vi "通信并与其他模块交互 (子VI).vi"() -> ()   [LabVIEW 2016, in "质控单元.lvlib"]
uses:
  <vilib>/Plasmionique/MB Master/MB_Master_TCP/MB_Master_TCP.lvclass
  C:/Program Files (x86)/National Instruments/LabVIEW 2016/vi.lib/Plasmionique/MB Master/MB_Master/MB_Master.lvclass
  <vilib>/Plasmionique/MB Master/MB_Master/MB_Master.lvclass
  <vilib>/Plasmionique/MB Master/MB Master.lvlib
  <vilib>/Utility/config.llb/NI_LVConfig.lvlib
panel:
  out "CODCr测量状态":u16[](array[numeric])
  out "CODMn测量状态":u16[](array[numeric])
  out "总氮测量状态":u16[](array[numeric])
  out "总磷测量状态":u16[](array[numeric])
  out "氨氮测量状态":u16[](array[numeric])
  out "通讯状态":bool
  out "待处理插入数量":i32
  out "元素":cluster{"命令":string}[](array[cluster])
  out "队列中元素数量":i32
  in  "starting address 6":u16
  in  "values 6":u16[](array[numeric])
  in  "starting address 5":u16
  in  "values 5":u16[](array[numeric])
  in  "starting address 4":u16
  in  "values 4":u16[](array[numeric])
  in  "starting address 3":u16
  in  "values 3":u16[](array[numeric])
  in  "starting address 2":u16
  in  "values 2":u16[](array[numeric])
  in  "values":u16[](array[numeric])
  in  "starting address":u16
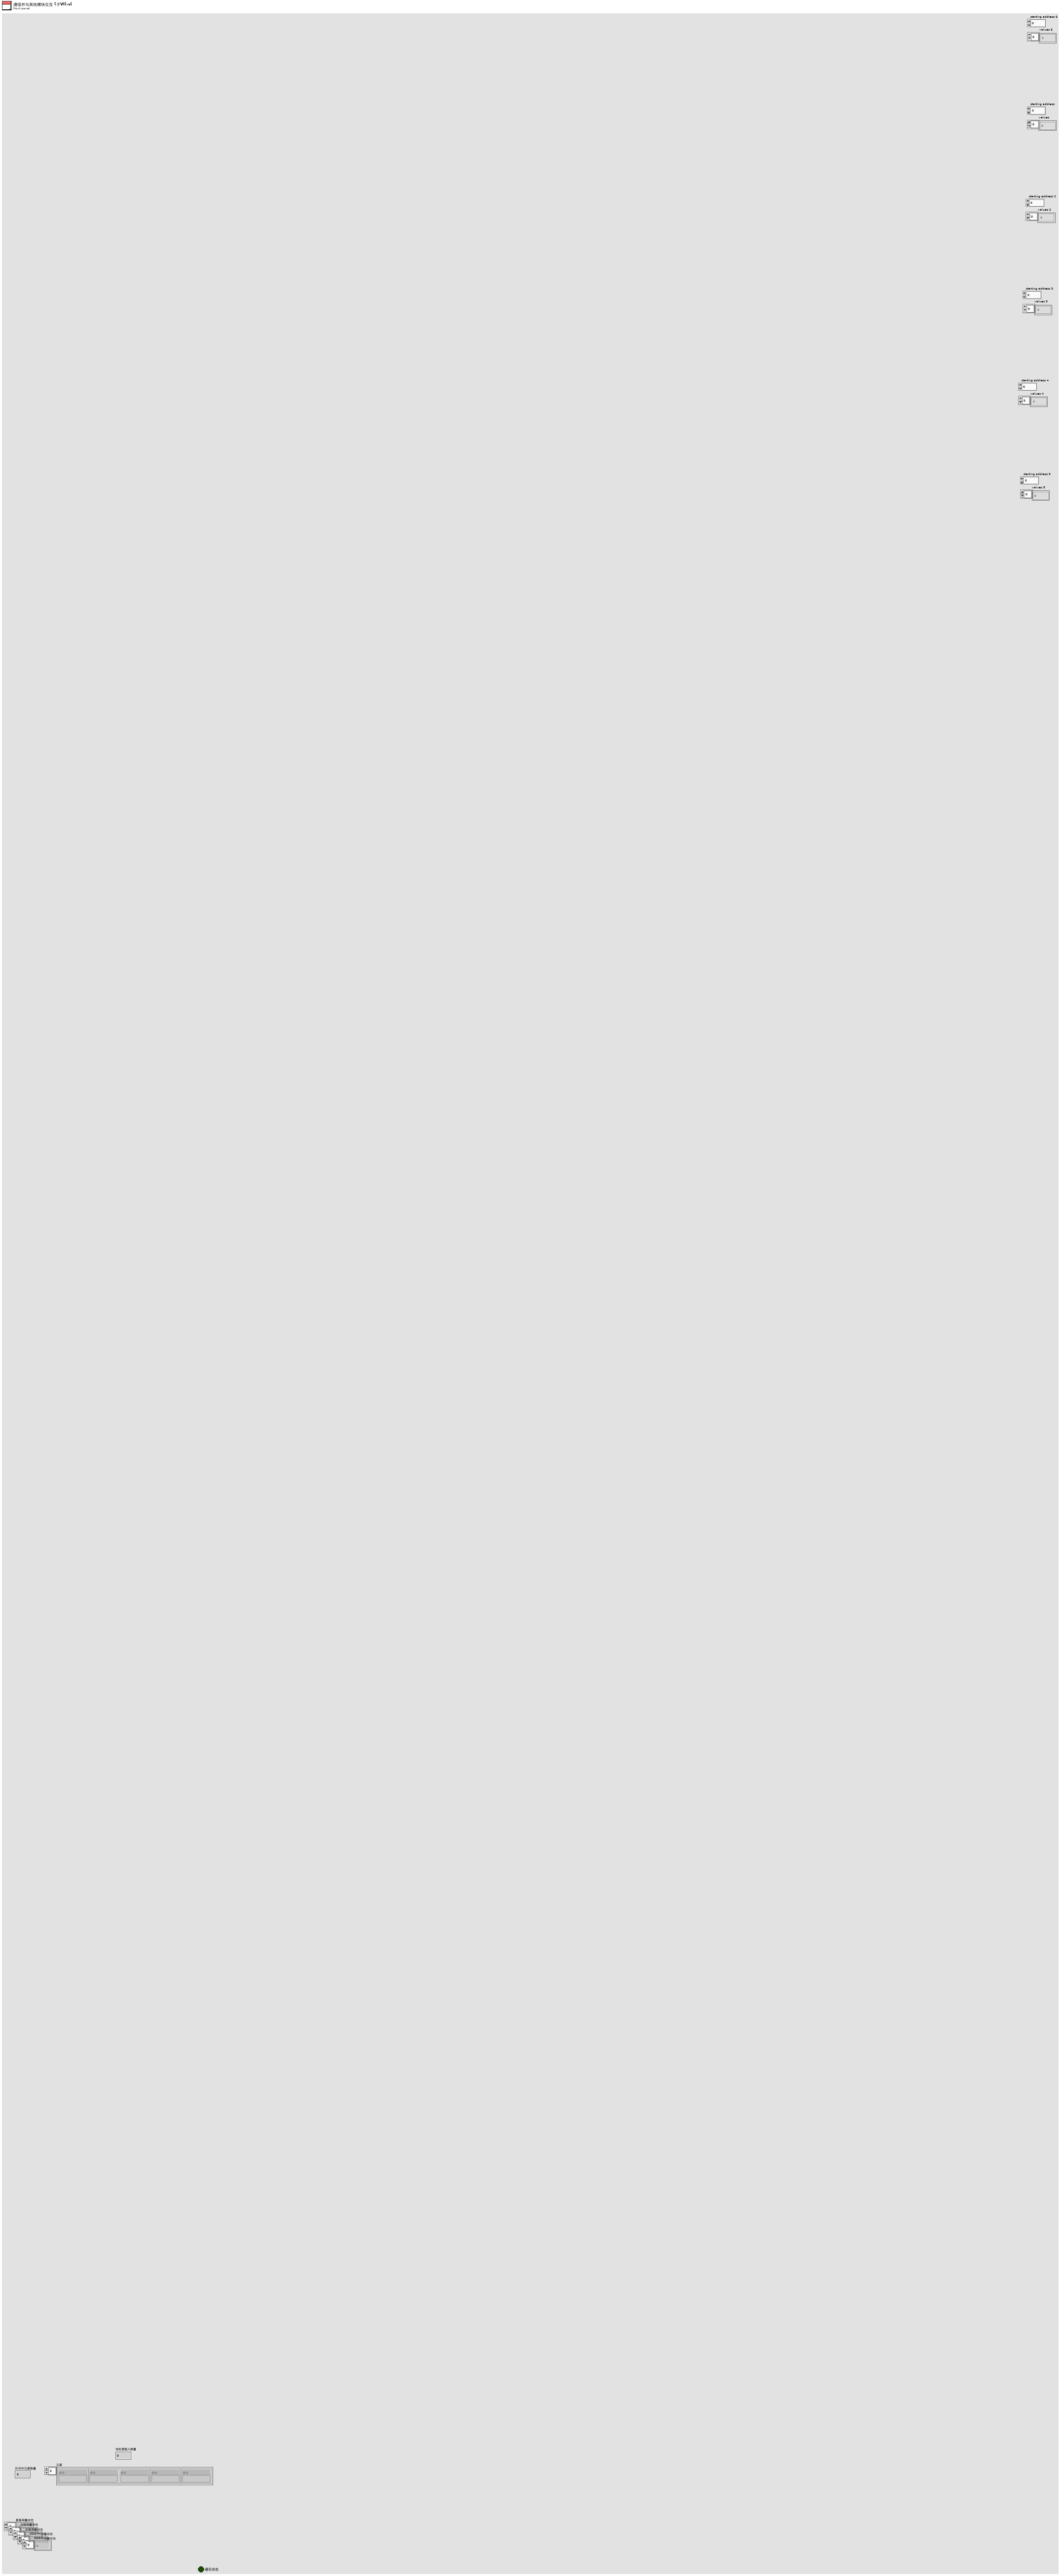
[diagram p1: front panel]
types:
  T1 = typedef "NI_LVConfig.lvlib/Config Data RefNum.ctl" = refnum<k1>
  T2 = cluster{"因子编码":u32, "单位":u16, "标样参考值":sgl, "水样数据时间":timestamp, "水样实测值":sgl, "水样数据标识":string, "标样数据时间":timestamp, "标样实测值":sgl, "标样数据标识":string, "空白数据时间":timestamp, "空白实测值":sgl, "空白数据标识":string, "零点核查数据时间":timestamp, "零点核查实测值":sgl, "零点核查数据标识":string, "跨度核查数据时间":timestamp, "跨度核查实测值":sgl, "跨度核查数据标识":string, "加标回收数据时间":timestamp, "加标回收实测值":sgl, "加标回收数据标识":string, "平行样数据时间":timestamp, "平行样实测值":sgl, "平行样数据标识":string}
  T3 = cluster{"系统时间":timestamp, "工作状态":enum16{"空闲", "水样测试", "标样核查", "零点核查", "跨度核查", "空白测试", "平行样测试", "加标回收", "空白校准", "标样校准", "初始化（清洗）"}, "测量模式":enum16{"待机", "连续模式", "周期模式", "定点模式", "受控模式", "手动模式"}, "告警代码":enum16{"无告警", "缺试剂告警", "缺水样告警", "缺蒸馏水告警", "缺标液告警", "仪表漏液告警", "标定异常告警", "超量程告警", "加热异常", "低试剂预警", "超上限告警", "超下限告警", "仪表内部其他异常", "滴定异常告警", "电极异常告警", "量程切换告警", "参数设置告警", "PH电极电位异常", "电导率电极异常", "浊度光度异常", "溶解氧电极异常", "溶解氧光强异常", "温度异常告警", "PH异常告警", "溶解氧异常告警", "电导率异常告警", "浊度异常告警", "叶绿素异常告警", "藻密度异常告警", "蓝绿藻异常告警", "ORP异常告警", "氨氮异常告警", "清洁刷异常告警", "SD卡异常告警", "蓝牙异常告警", "Wifi异常告警", "流程异常告警"}, "故障代码":enum16{"无故障", "电机故障", "温度故障", "通讯故障", "滴定故障"}, "日志代码":u16, "软件版本":u16, "F0":sgl, "F1":sgl, "F2":sgl, "F3":sgl, "T":sgl, "H":sgl, "id":u16, "flowid":u16, "量程":u16, "总磷控温温度1":sgl, "营养盐控温温度2":sgl, "ADC":sgl}
  T4 = cluster{"Registers[0]":u16, "Registers[1]":u16, "Registers[2]":u16, "Registers[3]":u16, "Registers[4]":u16, "Registers[5]":u16, "Registers[6]":u16, "Registers[7]":u16, "Registers[8]":u16, "Registers[9]":u16, "Registers[10]":u16, "Registers[11]":u16, "Registers[12]":u16, "Registers[13]":u16, "Registers[14]":u16, "Registers[15]":u16, "Registers[16]":u16, "Registers[17]":u16, "Registers[18]":u16, "Registers[19]":u16, "Registers[20]":u16, "Registers[21]":u16, "Registers[22]":u16, "Registers[23]":u16, "Registers[24]":u16, "Registers[25]":u16, "Registers[26]":u16, "Registers[27]":u16, "Registers[28]":u16, "Registers[29]":u16, "Registers[30]":u16, "Registers[31]":u16, "Registers[32]":u16, "Registers[33]":u16, "Registers[34]":u16, "Registers[35]":u16, "Registers[36]":u16, "Registers[37]":u16, "Registers[38]":u16, "Registers[39]":u16, "Registers[40]":u16, "Registers[41]":u16, "Registers[42]":u16, "Registers[43]":u16, "Registers[44]":u16, "Registers[45]":u16, "Registers[46]":u16, "Registers[47]":u16, "Registers[48]":u16, "Registers[49]":u16, "Registers[50]":u16, "Registers[51]":u16, "Registers[52]":u16, "Registers[53]":u16, "Registers[54]":u16, "Registers[55]":u16, "Registers[56]":u16}
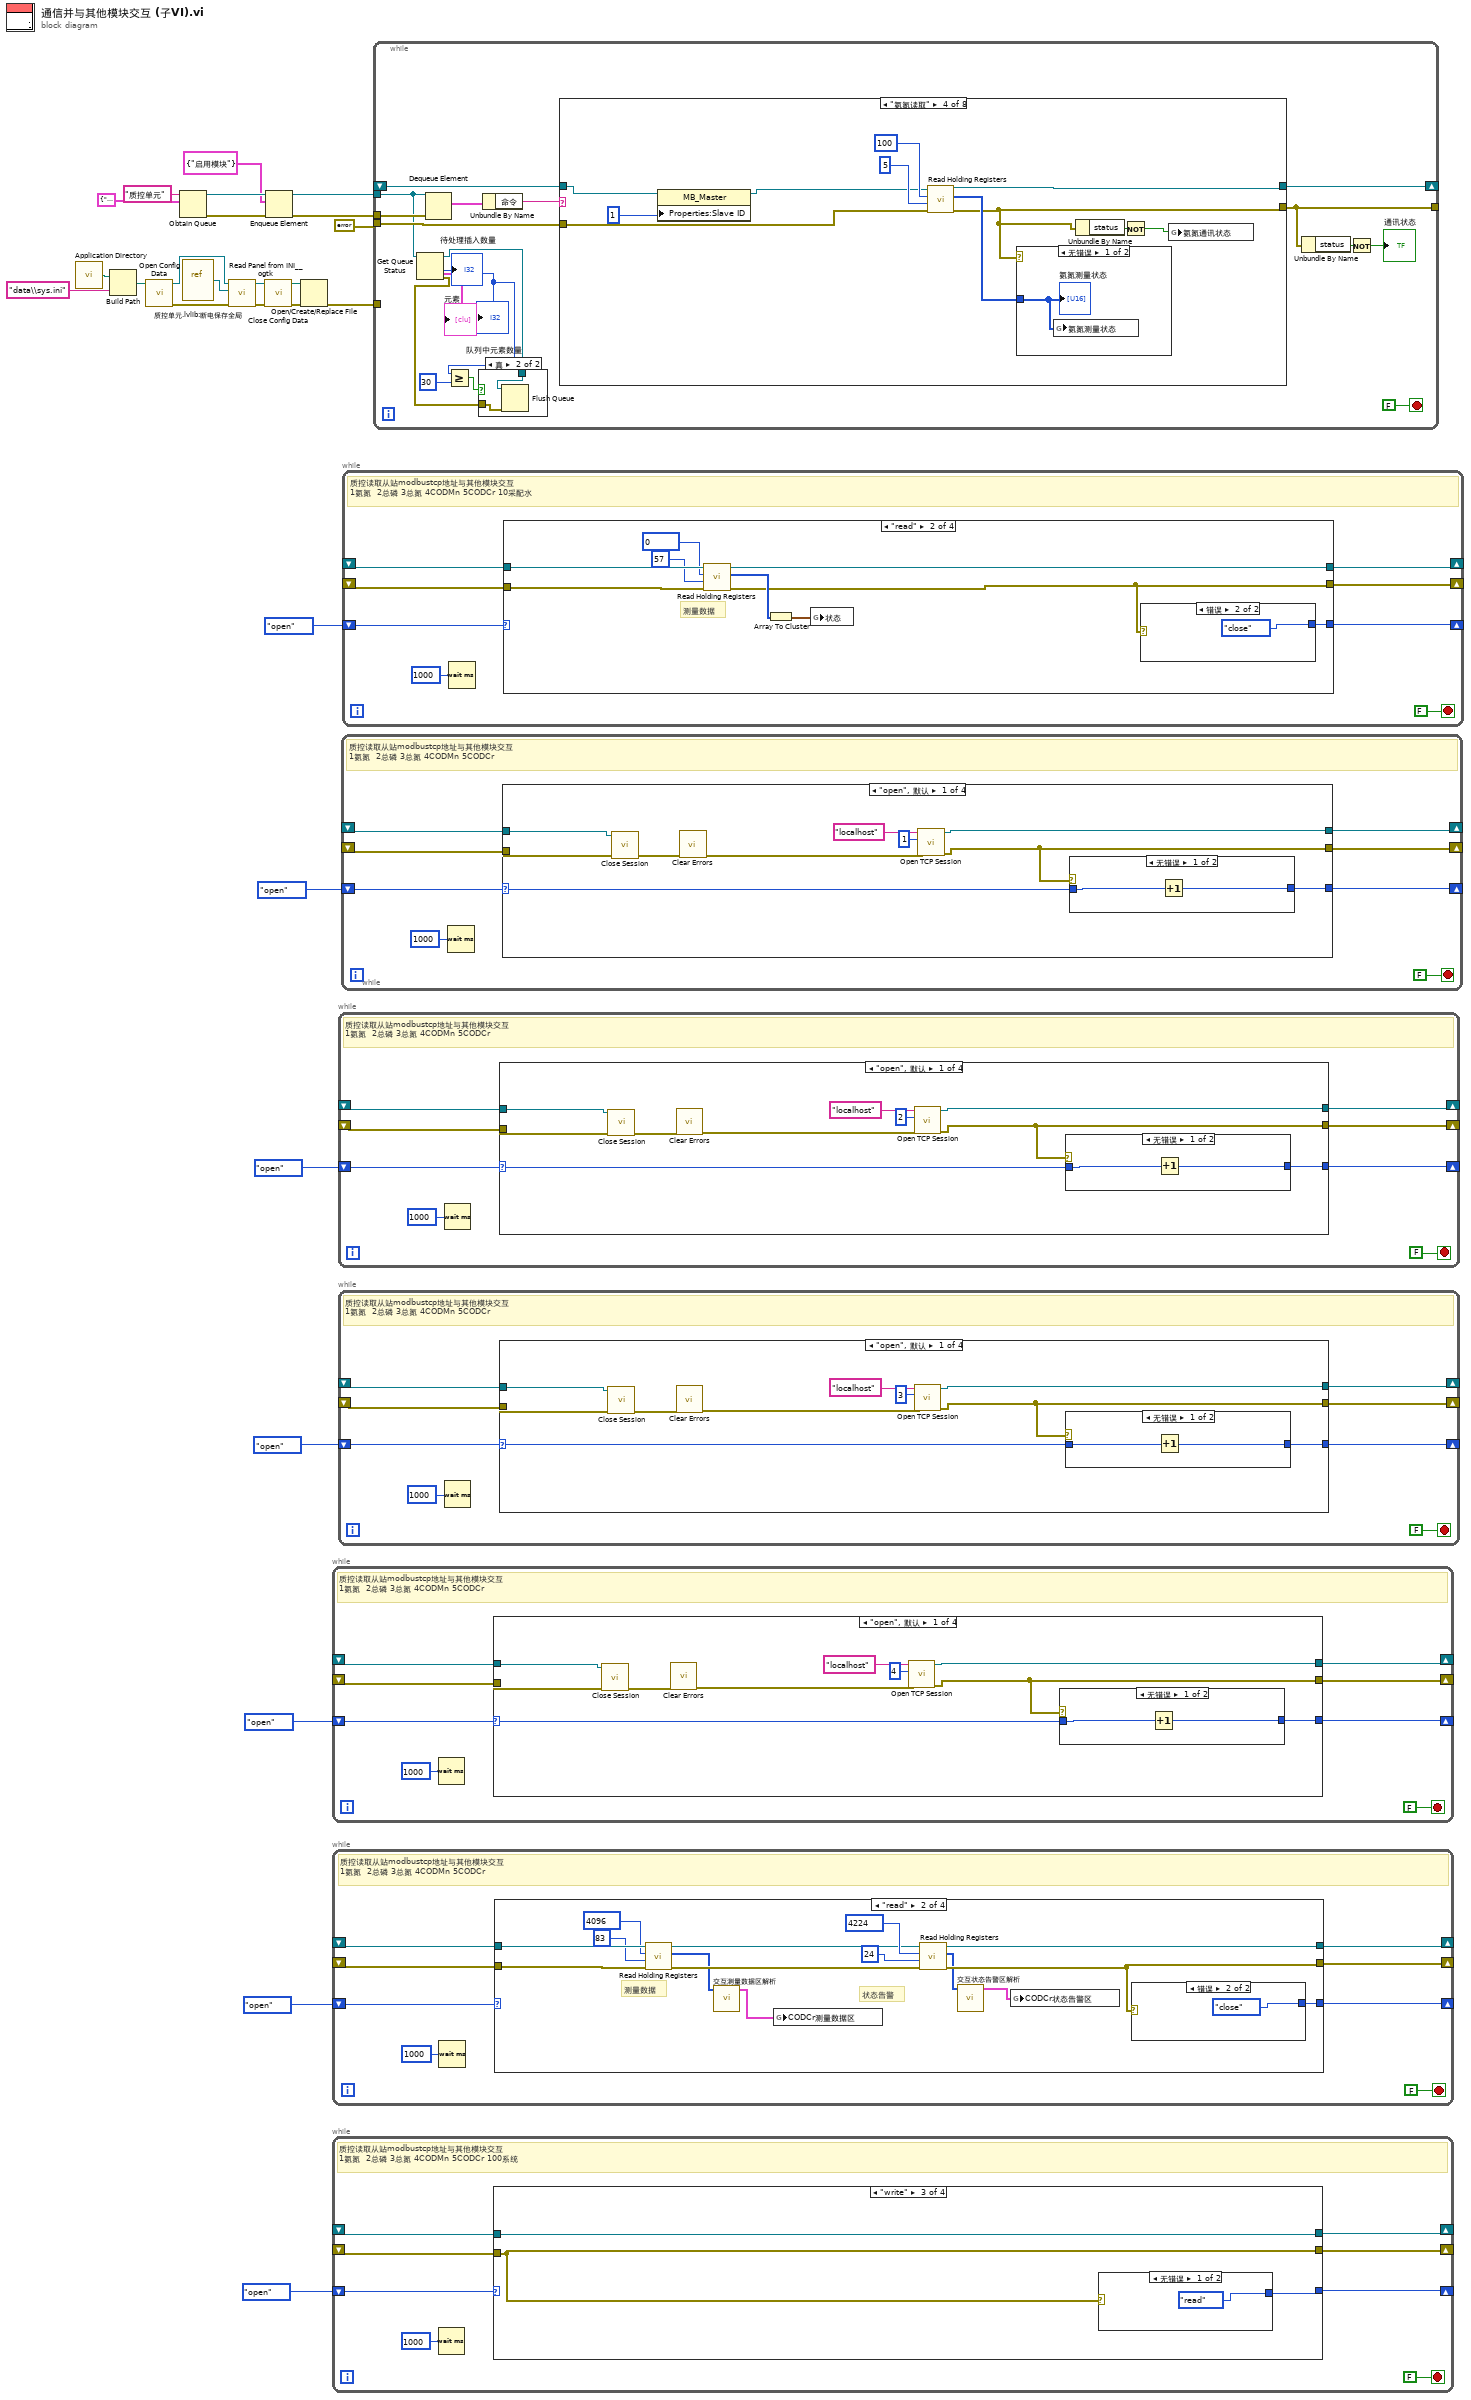
[diagram p0: block diagram]
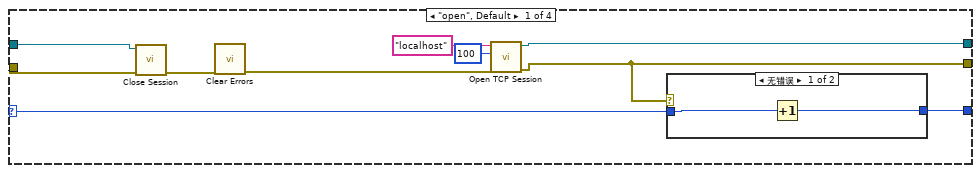
[diagram p2: hidden frame]
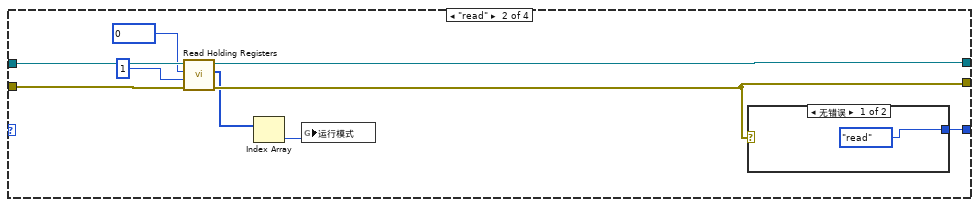
[diagram p4: hidden frame]
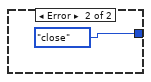
[diagram p5: hidden frame]
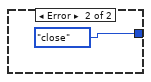
[diagram p6: hidden frame]
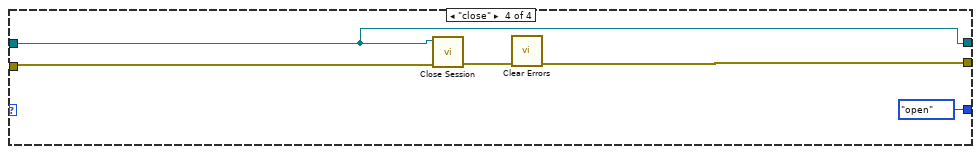
[diagram p7: hidden frame]
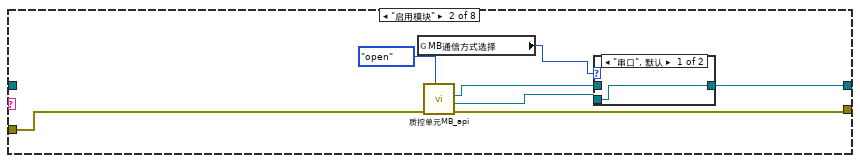
[diagram p10: hidden frame]
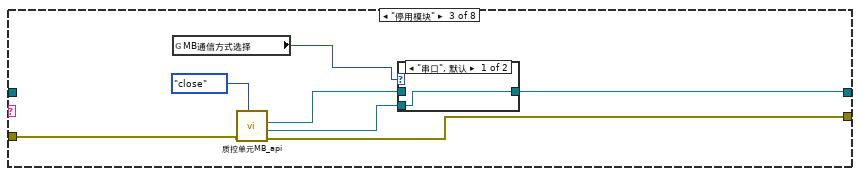
[diagram p12: hidden frame]
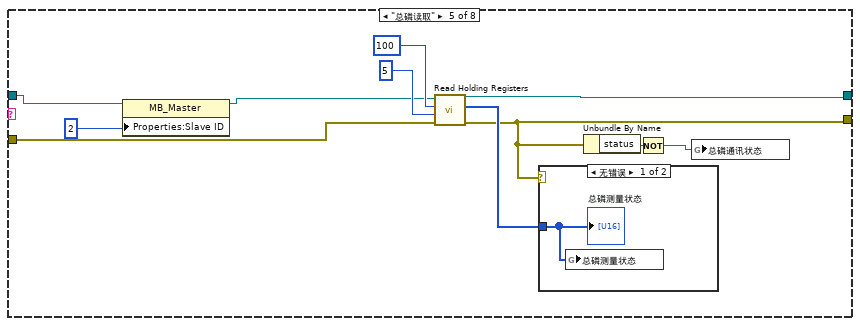
[diagram p15: hidden frame]
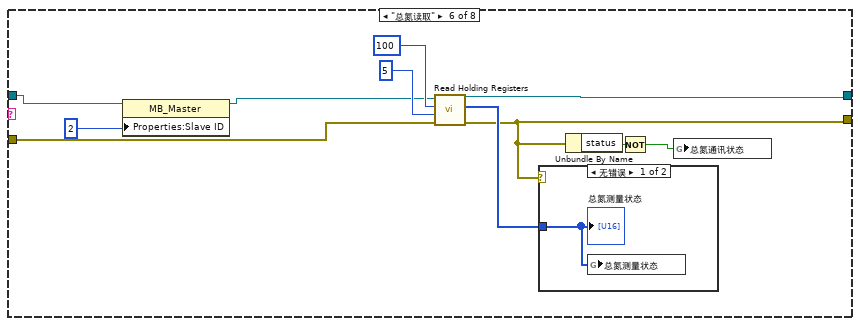
[diagram p17: hidden frame]
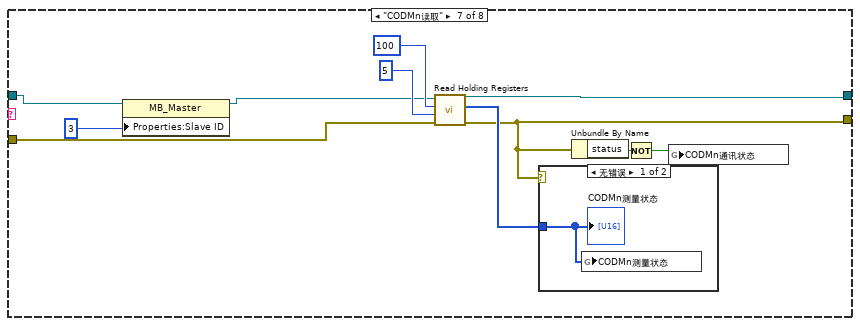
[diagram p19: hidden frame]
diagram:
  n1 = call <vilib>:"Application Directory.vi"() -> ("Application Directory"=w14:path)
  n2 = Build Path(base path=w14, name or relative path="data\\sys.ini" ("名称或相对路径")) -> (appended path=w12:path)
  n3 = call <vilib>:"Open Config Data.vi"("configuration file path"=w12) -> ("error out"=w8:errorcluster, "refnum"=w11:T1)  [unwired: 8 in, 1 out]
  n4 = Obtain Queue(name (unnamed)="质控单元" ("名称（未命名）"), element data type=cluster{"命令":string} {"命令"="启用模块"} ("元素")) -> (queue out=w17:refnum<queue>, error out=w16:errorcluster)  [unwired: 3 in, 1 out]
  n5 = vi-ref "质控单元.lvlib:断电保存全局.vi"() -> (w10:refnum<vi>)
  n6 = call <userlib>:"Read Panel from INI__ogtk.vi"("error in (no error)"=w8, "VI ref"=w10, "refnum"=w11) -> ("error out"=w7:errorcluster, "refnum out"=w9:T1)  [unwired: 7 in]
  n7 = call <vilib>:"Close Config Data.vi"("error in (no error)"=w7, "refnum"=w9) -> ("error out"=w6:errorcluster, "file path"=w5:path)  [unwired: 8 in]
  n8 = Enqueue Element(queue=w17, element=cluster{"命令":string} {"命令"="启用模块"} ("元素"), error in (no error)=w16) -> (queue out=w3:refnum<queue>, error out=w2:errorcluster)  [unwired: 1 in, 1 out]
  n9 = Open/Create/Replace File(file path (use dialog)=w5, error in=w6) -> (error out=w4:errorcluster)  [unwired: 4 in, 2 out]
  n10 = while {
    shift-right: [w32] -> _
    shift-left: _ -> [w34]
    shift-right: [w31] -> _
    shift-left: _ -> [w33]
    shift-right: [w28] -> _
    shift-left: enum16{"open", "read", "write", "close"}."open" -> [w29]
    stop <- FALSE stop-if-true
    # "质控读取从站modbustcp地址与其他模块交互\n1氨氮  2总磷 3总氮 4CODMn 5CODCr"
    n11 = Wait (ms)(milliseconds to wait=u32 1000 ("等待时间（毫秒）")) -> ()  [unwired: 1 out]
    n12 = case shown="\"open\", 默认" w29 {
      selector: w29 -> [w36 _ _ _]
      tunnel: w34 -> [w41 w72 w80 w88]
      tunnel: w33 -> [w40 w69 w79 w87]
      tunnel: [w42 w67 w78 w88] -> w32
      tunnel: [w37 w66 w77 w85] -> w31
      tunnel: [w35 w68 w81 enum16{"open", "read", "write", "close"}."open"] -> w28
      frame "open", Default {
        n13 = call-dynamic "Close Session.vi"("error in (no error)"=w40, "MB session in"=w41) -> ("error out"=w39:errorcluster)  [unwired: 9 in]
        n14 = call <vilib>:"Clear Errors.vi"("error in (no error)"=w39) -> ("error out"=w38:errorcluster)  [unwired: 5 in, 1 out]
        n15 = call <vilib>:"Open TCP Session.vi"("error in (no error)"=w38, "Port (502)"=u16 4, "IP Address"="localhost") -> ("error out"=w37:errorcluster, "MB_TCP session"=w42:refnum<class "MB_Master_TCP.lvclass">)  [unwired: 7 in]
        n16 = case shown="无错误" w37 {
          tunnel: w36 -> [w46 w47]
          tunnel: [w45 w47] -> w35
          frame No Error {
            n17 = Increment(x=w46) -> (x+1=w45:enum16{"open", "read", "write", "close"})
          }
          frame Error {
          }
        }
      }
      frame "read" {
        # "测量数据"
        n18 = call <vilib>:"Read Holding Registers.vi"("error in (no error)"=w69, "quantity"=u16 30, "starting address"=u16 0, "MB session in"=w72) -> ("error out"=w66:errorcluster, "Registers"=w65:u16[], "MB session out"=w67:refnum<class "MB_Master.lvclass">)  [unwired: 5 in]
        n19 = Index Array(array=w65) -> (element #1=w64:u16, element #2=w63:u16, element #3=w62:u16, element #4=w58:u16, element #5=w57:u16, element #6=w56:u16, element #7=w55:u16, element #8=w53:u16, element #9=w52:u16, element #10=w51:u16)  [unwired: 10 in]
        n20 = Build Array(w63, w62) -> (w61:u16[])
        n21 = Build Array(w57, w56, w55, w53, w52, w51) -> (w54:u16[])
        n22 = call "HexToDate.vi"("数组"=w54) -> ("DATE"=w50:timestamp[])  [unwired: 10 in]
        n23 = call "HexToCDABFloat.vi"("数组"=w61) -> ("FLOAT"=w60:sgl[])  [unwired: 10 in]
        n24 = Index Array(array=w50) -> (element #1=w49:timestamp, element #2=w48:timestamp)  [unwired: 2 in]
        n25 = Index Array(array=w60) -> (element=w59:sgl)  [unwired: 1 in]
        n26 = global write "与CODMn交互全局.vi" "COD浓度（mg/L)"(w59) -> ()
        n27 = global write "与CODMn交互全局.vi" "加标回收启动时间"(w49) -> ()
        n28 = global write "与CODMn交互全局.vi" "CODMn工作状态"(w64) -> ()
        n29 = global write "与CODMn交互全局.vi" "水样启动时间"(w48) -> ()
        n30 = global write "与CODMn交互全局.vi" "多列列表框"(w58) -> ()
        n31 = case shown="错误" w66 {
          tunnel: [enum16{"open", "read", "write", "close"}."read" enum16{"open", "read", "write", "close"}."close"] -> w68
          frame No Error {
          }
          frame Error {
          }
        }
      }
      frame "write" {
        n32 = call <vilib>:"Write Multiple Registers.vi"("error in (no error)"=w79, "values"="values 4", "starting address"="starting address 4", "MB session in"=w80) -> ("error out"=w77:errorcluster, "MB session out"=w78:refnum<class "MB_Master.lvclass">)  [unwired: 6 in]
        n33 = case shown="错误" w77 {
          tunnel: [enum16{"open", "read", "write", "close"}."read" enum16{"open", "read", "write", "close"}."close"] -> w81
          frame No Error {
          }
          frame Error {
          }
        }
      }
      frame "close" {
        n34 = call-dynamic "Close Session.vi"("error in (no error)"=w87, "MB session in"=w88) -> ("error out"=w86:errorcluster)  [unwired: 9 in]
        n35 = call <vilib>:"Clear Errors.vi"("error in (no error)"=w86) -> ("error out"=w85:errorcluster)  [unwired: 5 in, 1 out]
      }
    }
  }
  n36 = while {
    shift-right: [w94] -> _
    shift-left: _ -> [w96]
    shift-right: [w93] -> _
    shift-left: _ -> [w95]
    shift-right: [w90] -> _
    shift-left: enum16{"open", "read", "write", "close"}."open" -> [w91]
    stop <- FALSE stop-if-true
    # "质控读取从站modbustcp地址与其他模块交互\n1氨氮  2总磷 3总氮 4CODMn 5CODCr 100系统"
    n37 = Wait (ms)(milliseconds to wait=u32 1000 ("等待时间（毫秒）")) -> ()  [unwired: 1 out]
    n38 = case shown="\"write\"" w91 {
      selector: w91 -> [w98 _ _ _]
      tunnel: w96 -> [w103 w118 w122 w130]
      tunnel: w95 -> [w102 w115 w121 w129]
      tunnel: [w104 w113 w122 w130] -> w94
      tunnel: [w99 w112 w121 w127] -> w93
      tunnel: [w97 w114 w123 enum16{"open", "read", "write", "close"}."open"] -> w90
      frame "open", Default {
        n39 = call-dynamic "Close Session.vi"("error in (no error)"=w102, "MB session in"=w103) -> ("error out"=w101:errorcluster)  [unwired: 9 in]
        n40 = call <vilib>:"Clear Errors.vi"("error in (no error)"=w101) -> ("error out"=w100:errorcluster)  [unwired: 5 in, 1 out]
        n41 = call <vilib>:"Open TCP Session.vi"("error in (no error)"=w100, "Port (502)"=u16 100, "IP Address"="localhost") -> ("error out"=w99:errorcluster, "MB_TCP session"=w104:refnum<class "MB_Master_TCP.lvclass">)  [unwired: 7 in]
        n42 = case shown="无错误" w99 {
          tunnel: w98 -> [w108 w109]
          tunnel: [w107 w109] -> w97
          frame No Error {
            n43 = Increment(x=w108) -> (x+1=w107:enum16{"open", "read", "write", "close"})
          }
          frame Error {
          }
        }
      }
      frame "read" {
        n44 = call <vilib>:"Read Holding Registers.vi"("error in (no error)"=w115, "quantity"=u16 1, "starting address"=u16 0, "MB session in"=w118) -> ("error out"=w112:errorcluster, "Registers"=w111:u16[], "MB session out"=w113:refnum<class "MB_Master.lvclass">)  [unwired: 5 in]
        n45 = Index Array(array=w111) -> (element=w110:u16)  [unwired: 1 in]
        n46 = global write "系统交互.vi" "运行模式"(w110) -> ()
        n47 = case shown="无错误" w112 {
          tunnel: [enum16{"open", "read", "write", "close"}."read" enum16{"open", "read", "write", "close"}."close"] -> w114
          frame No Error {
          }
          frame Error {
          }
        }
      }
      frame "write" {
        n48 = case shown="无错误" w121 {
          tunnel: [enum16{"open", "read", "write", "close"}."read" enum16{"open", "read", "write", "close"}."close"] -> w123
          frame No Error {
          }
          frame Error {
          }
        }
      }
      frame "close" {
        n49 = call-dynamic "Close Session.vi"("error in (no error)"=w129, "MB session in"=w130) -> ("error out"=w128:errorcluster)  [unwired: 9 in]
        n50 = call <vilib>:"Clear Errors.vi"("error in (no error)"=w128) -> ("error out"=w127:errorcluster)  [unwired: 5 in, 1 out]
      }
    }
  }
  n51 = while {
    shift-right: [w136] -> _
    shift-left: _ -> [w138]
    shift-right: [w135] -> _
    shift-left: _ -> [w137]
    shift-right: [w132] -> _
    shift-left: enum16{"open", "read", "write", "close"}."open" -> [w133]
    stop <- FALSE stop-if-true
    # "质控读取从站modbustcp地址与其他模块交互\n1氨氮  2总磷 3总氮 4CODMn 5CODCr"
    n52 = Wait (ms)(milliseconds to wait=u32 1000 ("等待时间（毫秒）")) -> ()  [unwired: 1 out]
    n53 = case shown="\"read\"" w133 {
      selector: w133 -> [w140 _ _ _]
      tunnel: w138 -> [w145 w166 w174 w182]
      tunnel: w137 -> [w144 w163 w173 w181]
      tunnel: [w146 w157 w172 w182] -> w136
      tunnel: [w141 w156 w171 w179] -> w135
      tunnel: [w139 w162 w175 enum16{"open", "read", "write", "close"}."open"] -> w132
      frame "open", Default {
        n54 = call-dynamic "Close Session.vi"("error in (no error)"=w144, "MB session in"=w145) -> ("error out"=w143:errorcluster)  [unwired: 9 in]
        n55 = call <vilib>:"Clear Errors.vi"("error in (no error)"=w143) -> ("error out"=w142:errorcluster)  [unwired: 5 in, 1 out]
        n56 = call <vilib>:"Open TCP Session.vi"("error in (no error)"=w142, "Port (502)"=u16 5, "IP Address"="localhost") -> ("error out"=w141:errorcluster, "MB_TCP session"=w146:refnum<class "MB_Master_TCP.lvclass">)  [unwired: 7 in]
        n57 = case shown="无错误" w141 {
          tunnel: w140 -> [w150 w151]
          tunnel: [w149 w151] -> w139
          frame No Error {
            n58 = Increment(x=w150) -> (x+1=w149:enum16{"open", "read", "write", "close"})
          }
          frame Error {
          }
        }
      }
      frame "read" {
        # "状态告警"
        # "测量数据"
        n59 = call <vilib>:"Read Holding Registers.vi"("error in (no error)"=w163, "quantity"=u16 83, "starting address"=u16 4096, "MB session in"=w166) -> ("error out"=w158:errorcluster, "Registers"=w155:u16[], "MB session out"=w159:refnum<class "MB_Master.lvclass">)  [unwired: 5 in]
        n60 = call "交互测量数据区解析.vi"("数组"=w155) -> ("测量数据区"=w153:T2)  [unwired: 10 in]
        n61 = global write "与CODCr交互全局.vi" "CODCr测量数据区"(w153) -> ()
        n62 = call <vilib>:"Read Holding Registers.vi"("error in (no error)"=w158, "quantity"=u16 24, "starting address"=u16 4224, "MB session in"=w159) -> ("error out"=w156:errorcluster, "Registers"=w154:u16[], "MB session out"=w157:refnum<class "MB_Master.lvclass">)  [unwired: 5 in]
        n63 = call "交互状态告警区解析.vi"("数组"=w154) -> ("状态告警区"=w152:T3)  [unwired: 10 in]
        n64 = global write "与CODCr交互全局.vi" "CODCr状态告警区"(w152) -> ()
        n65 = case shown="错误" w156 {
          tunnel: [enum16{"open", "read", "write", "close"}."read" enum16{"open", "read", "write", "close"}."close"] -> w162
          frame No Error {
          }
          frame Error {
          }
        }
      }
      frame "write" {
        n66 = call <vilib>:"Write Multiple Registers.vi"("error in (no error)"=w173, "values"="values 5", "starting address"="starting address 5", "MB session in"=w174) -> ("error out"=w171:errorcluster, "MB session out"=w172:refnum<class "MB_Master.lvclass">)  [unwired: 6 in]
        n67 = case shown="错误" w171 {
          tunnel: [enum16{"open", "read", "write", "close"}."read" enum16{"open", "read", "write", "close"}."close"] -> w175
          frame No Error {
          }
          frame Error {
          }
        }
      }
      frame "close" {
        n68 = call-dynamic "Close Session.vi"("error in (no error)"=w181, "MB session in"=w182) -> ("error out"=w180:errorcluster)  [unwired: 9 in]
        n69 = call <vilib>:"Clear Errors.vi"("error in (no error)"=w180) -> ("error out"=w179:errorcluster)  [unwired: 5 in, 1 out]
      }
    }
  }
  n70 = while {
    shift-right: [w188] -> _
    shift-left: _ -> [w190]
    shift-right: [w187] -> _
    shift-left: _ -> [w189]
    shift-right: [w184] -> _
    shift-left: enum16{"open", "read", "write", "close"}."open" -> [w185]
    stop <- FALSE stop-if-true
    # "质控读取从站modbustcp地址与其他模块交互\n1氨氮  2总磷 3总氮 4CODMn 5CODCr"
    n71 = Wait (ms)(milliseconds to wait=u32 1000 ("等待时间（毫秒）")) -> ()  [unwired: 1 out]
    n72 = case shown="\"open\", 默认" w185 {
      selector: w185 -> [w192 _ _ _]
      tunnel: w190 -> [w197 w218 w226 w234]
      tunnel: w189 -> [w196 w215 w225 w233]
      tunnel: [w198 w209 w224 w234] -> w188
      tunnel: [w193 w208 w223 w231] -> w187
      tunnel: [w191 w214 w227 enum16{"open", "read", "write", "close"}."open"] -> w184
      frame "open", Default {
        n73 = call-dynamic "Close Session.vi"("error in (no error)"=w196, "MB session in"=w197) -> ("error out"=w195:errorcluster)  [unwired: 9 in]
        n74 = call <vilib>:"Clear Errors.vi"("error in (no error)"=w195) -> ("error out"=w194:errorcluster)  [unwired: 5 in, 1 out]
        n75 = call <vilib>:"Open TCP Session.vi"("error in (no error)"=w194, "Port (502)"=u16 2, "IP Address"="localhost") -> ("error out"=w193:errorcluster, "MB_TCP session"=w198:refnum<class "MB_Master_TCP.lvclass">)  [unwired: 7 in]
        n76 = case shown="无错误" w193 {
          tunnel: w192 -> [w202 w203]
          tunnel: [w201 w203] -> w191
          frame No Error {
            n77 = Increment(x=w202) -> (x+1=w201:enum16{"open", "read", "write", "close"})
          }
          frame Error {
          }
        }
      }
      frame "read" {
        # "状态告警"
        # "测量数据"
        n78 = call <vilib>:"Read Holding Registers.vi"("error in (no error)"=w215, "quantity"=u16 83, "starting address"=u16 4096, "MB session in"=w218) -> ("error out"=w210:errorcluster, "Registers"=w207:u16[], "MB session out"=w211:refnum<class "MB_Master.lvclass">)  [unwired: 5 in]
        n79 = call "交互测量数据区解析.vi"("数组"=w207) -> ("测量数据区"=w205:T2)  [unwired: 10 in]
        n80 = global write "与总磷交互全局.vi" "总磷测量数据区"(w205) -> ()
        n81 = call <vilib>:"Read Holding Registers.vi"("error in (no error)"=w210, "quantity"=u16 24, "starting address"=u16 4224, "MB session in"=w211) -> ("error out"=w208:errorcluster, "Registers"=w206:u16[], "MB session out"=w209:refnum<class "MB_Master.lvclass">)  [unwired: 5 in]
        n82 = call "交互状态告警区解析.vi"("数组"=w206) -> ("状态告警区"=w204:T3)  [unwired: 10 in]
        n83 = global write "与总磷交互全局.vi" "总磷状态告警区"(w204) -> ()
        n84 = case shown="错误" w208 {
          tunnel: [enum16{"open", "read", "write", "close"}."read" enum16{"open", "read", "write", "close"}."close"] -> w214
          frame No Error {
          }
          frame Error {
          }
        }
      }
      frame "write" {
        n85 = call <vilib>:"Write Multiple Registers.vi"("error in (no error)"=w225, "values"="values 2", "starting address"="starting address 2", "MB session in"=w226) -> ("error out"=w223:errorcluster, "MB session out"=w224:refnum<class "MB_Master.lvclass">)  [unwired: 6 in]
        n86 = case shown="错误" w223 {
          tunnel: [enum16{"open", "read", "write", "close"}."read" enum16{"open", "read", "write", "close"}."close"] -> w227
          frame No Error {
          }
          frame Error {
          }
        }
      }
      frame "close" {
        n87 = call-dynamic "Close Session.vi"("error in (no error)"=w233, "MB session in"=w234) -> ("error out"=w232:errorcluster)  [unwired: 9 in]
        n88 = call <vilib>:"Clear Errors.vi"("error in (no error)"=w232) -> ("error out"=w231:errorcluster)  [unwired: 5 in, 1 out]
      }
    }
  }
  n89 = while {
    shift-right: [w240] -> _
    shift-left: _ -> [w242]
    shift-right: [w239] -> _
    shift-left: _ -> [w241]
    shift-right: [w236] -> _
    shift-left: enum16{"open", "read", "write", "close"}."open" -> [w237]
    stop <- FALSE stop-if-true
    # "质控读取从站modbustcp地址与其他模块交互\n1氨氮  2总磷 3总氮 4CODMn 5CODCr"
    n90 = Wait (ms)(milliseconds to wait=u32 1000 ("等待时间（毫秒）")) -> ()  [unwired: 1 out]
    n91 = case shown="\"open\", 默认" w237 {
      selector: w237 -> [w244 _ _ _]
      tunnel: w242 -> [w249 w270 w278 w286]
      tunnel: w241 -> [w248 w267 w277 w285]
      tunnel: [w250 w261 w276 w286] -> w240
      tunnel: [w245 w260 w275 w283] -> w239
      tunnel: [w243 w266 w279 enum16{"open", "read", "write", "close"}."open"] -> w236
      frame "open", Default {
        n92 = call-dynamic "Close Session.vi"("error in (no error)"=w248, "MB session in"=w249) -> ("error out"=w247:errorcluster)  [unwired: 9 in]
        n93 = call <vilib>:"Clear Errors.vi"("error in (no error)"=w247) -> ("error out"=w246:errorcluster)  [unwired: 5 in, 1 out]
        n94 = call <vilib>:"Open TCP Session.vi"("error in (no error)"=w246, "Port (502)"=u16 3, "IP Address"="localhost") -> ("error out"=w245:errorcluster, "MB_TCP session"=w250:refnum<class "MB_Master_TCP.lvclass">)  [unwired: 7 in]
        n95 = case shown="无错误" w245 {
          tunnel: w244 -> [w254 w255]
          tunnel: [w253 w255] -> w243
          frame No Error {
            n96 = Increment(x=w254) -> (x+1=w253:enum16{"open", "read", "write", "close"})
          }
          frame Error {
          }
        }
      }
      frame "read" {
        # "状态告警"
        # "测量数据"
        n97 = call <vilib>:"Read Holding Registers.vi"("error in (no error)"=w267, "quantity"=u16 83, "starting address"=u16 4096, "MB session in"=w270) -> ("error out"=w262:errorcluster, "Registers"=w259:u16[], "MB session out"=w263:refnum<class "MB_Master.lvclass">)  [unwired: 5 in]
        n98 = call "交互测量数据区解析.vi"("数组"=w259) -> ("测量数据区"=w257:T2)  [unwired: 10 in]
        n99 = global write "与总氮交互全局.vi" "总氮测量数据区"(w257) -> ()
        n100 = call <vilib>:"Read Holding Registers.vi"("error in (no error)"=w262, "quantity"=u16 24, "starting address"=u16 4224, "MB session in"=w263) -> ("error out"=w260:errorcluster, "Registers"=w258:u16[], "MB session out"=w261:refnum<class "MB_Master.lvclass">)  [unwired: 5 in]
        n101 = call "交互状态告警区解析.vi"("数组"=w258) -> ("状态告警区"=w256:T3)  [unwired: 10 in]
        n102 = global write "与总氮交互全局.vi" "总氮状态告警区"(w256) -> ()
        n103 = case shown="错误" w260 {
          tunnel: [enum16{"open", "read", "write", "close"}."read" enum16{"open", "read", "write", "close"}."close"] -> w266
          frame No Error {
          }
          frame Error {
          }
        }
      }
      frame "write" {
        n104 = call <vilib>:"Write Multiple Registers.vi"("error in (no error)"=w277, "values"="values 3", "starting address"="starting address 3", "MB session in"=w278) -> ("error out"=w275:errorcluster, "MB session out"=w276:refnum<class "MB_Master.lvclass">)  [unwired: 6 in]
        n105 = case shown="错误" w275 {
          tunnel: [enum16{"open", "read", "write", "close"}."read" enum16{"open", "read", "write", "close"}."close"] -> w279
          frame No Error {
          }
          frame Error {
          }
        }
      }
      frame "close" {
        n106 = call-dynamic "Close Session.vi"("error in (no error)"=w285, "MB session in"=w286) -> ("error out"=w284:errorcluster)  [unwired: 9 in]
        n107 = call <vilib>:"Clear Errors.vi"("error in (no error)"=w284) -> ("error out"=w283:errorcluster)  [unwired: 5 in, 1 out]
      }
    }
  }
  n108 = while {
    shift-right: [w292] -> _
    shift-left: _ -> [w294]
    shift-right: [w291] -> _
    shift-left: _ -> [w293]
    shift-right: [w288] -> _
    shift-left: enum16{"open", "read", "write", "close"}."open" -> [w289]
    stop <- FALSE stop-if-true
    # "质控读取从站modbustcp地址与其他模块交互\n1氨氮  2总磷 3总氮 4CODMn 5CODCr"
    n109 = Wait (ms)(milliseconds to wait=u32 1000 ("等待时间（毫秒）")) -> ()  [unwired: 1 out]
    n110 = case shown="\"open\", 默认" w289 {
      selector: w289 -> [w296 _ _ _]
      tunnel: w294 -> [w301 w322 w330 w338]
      tunnel: w293 -> [w300 w319 w329 w337]
      tunnel: [w302 w313 w328 w338] -> w292
      tunnel: [w297 w312 w327 w335] -> w291
      tunnel: [w295 w318 w331 enum16{"open", "read", "write", "close"}."open"] -> w288
      frame "open", Default {
        n111 = call-dynamic "Close Session.vi"("error in (no error)"=w300, "MB session in"=w301) -> ("error out"=w299:errorcluster)  [unwired: 9 in]
        n112 = call <vilib>:"Clear Errors.vi"("error in (no error)"=w299) -> ("error out"=w298:errorcluster)  [unwired: 5 in, 1 out]
        n113 = call <vilib>:"Open TCP Session.vi"("error in (no error)"=w298, "Port (502)"=u16 1, "IP Address"="localhost") -> ("error out"=w297:errorcluster, "MB_TCP session"=w302:refnum<class "MB_Master_TCP.lvclass">)  [unwired: 7 in]
        n114 = case shown="无错误" w297 {
          tunnel: w296 -> [w306 w307]
          tunnel: [w305 w307] -> w295
          frame No Error {
            n115 = Increment(x=w306) -> (x+1=w305:enum16{"open", "read", "write", "close"})
          }
          frame Error {
          }
        }
      }
      frame "read" {
        # "状态告警"
        # "测量数据"
        n116 = call <vilib>:"Read Holding Registers.vi"("error in (no error)"=w319, "quantity"=u16 83, "starting address"=u16 4096, "MB session in"=w322) -> ("error out"=w314:errorcluster, "Registers"=w311:u16[], "MB session out"=w315:refnum<class "MB_Master.lvclass">)  [unwired: 5 in]
        n117 = call "交互测量数据区解析.vi"("数组"=w311) -> ("测量数据区"=w310:T2)  [unwired: 10 in]
        n118 = global write "与氨氮交互全局.vi" "氨氮测量数据区"(w310) -> ()
        n119 = call <vilib>:"Read Holding Registers.vi"("error in (no error)"=w314, "quantity"=u16 24, "starting address"=u16 4224, "MB session in"=w315) -> ("error out"=w312:errorcluster, "Registers"=w309:u16[], "MB session out"=w313:refnum<class "MB_Master.lvclass">)  [unwired: 5 in]
        n120 = call "交互状态告警区解析.vi"("数组"=w309) -> ("状态告警区"=w308:T3)  [unwired: 10 in]
        n121 = global write "与氨氮交互全局.vi" "氨氮状态告警区"(w308) -> ()
        n122 = case shown="错误" w312 {
          tunnel: [enum16{"open", "read", "write", "close"}."read" enum16{"open", "read", "write", "close"}."close"] -> w318
          frame No Error {
          }
          frame Error {
          }
        }
      }
      frame "write" {
        n123 = call <vilib>:"Write Multiple Registers.vi"("error in (no error)"=w329, "values"="values", "starting address"="starting address", "MB session in"=w330) -> ("error out"=w327:errorcluster, "MB session out"=w328:refnum<class "MB_Master.lvclass">)  [unwired: 6 in]
        n124 = case shown="错误" w327 {
          tunnel: [enum16{"open", "read", "write", "close"}."read" enum16{"open", "read", "write", "close"}."close"] -> w331
          frame No Error {
          }
          frame Error {
          }
        }
      }
      frame "close" {
        n125 = call-dynamic "Close Session.vi"("error in (no error)"=w337, "MB session in"=w338) -> ("error out"=w336:errorcluster)  [unwired: 9 in]
        n126 = call <vilib>:"Clear Errors.vi"("error in (no error)"=w336) -> ("error out"=w335:errorcluster)  [unwired: 5 in, 1 out]
      }
    }
  }
  n127 = while {
    shift-right: [w344] -> _
    shift-left: _ -> [w346]
    shift-right: [w343] -> _
    shift-left: _ -> [w345]
    shift-right: [w340] -> _
    shift-left: enum16{"open", "read", "write", "close"}."open" -> [w341]
    stop <- FALSE stop-if-true
    # "质控读取从站modbustcp地址与其他模块交互\n1氨氮  2总磷 3总氮 4CODMn 5CODCr 10采配水"
    n128 = Wait (ms)(milliseconds to wait=u32 1000 ("等待时间（毫秒）")) -> ()  [unwired: 1 out]
    n129 = case shown="\"read\"" w341 {
      selector: w341 -> [w348 _ _ _]
      tunnel: w346 -> [w353 w368 w376 w384]
      tunnel: w345 -> [w352 w365 w375 w383]
      tunnel: [w354 w361 w374 w384] -> w344
      tunnel: [w349 w360 w373 w381] -> w343
      tunnel: [w347 w364 w377 enum16{"open", "read", "write", "close"}."open"] -> w340
      frame "open", Default {
        n130 = call-dynamic "Close Session.vi"("error in (no error)"=w352, "MB session in"=w353) -> ("error out"=w351:errorcluster)  [unwired: 9 in]
        n131 = call <vilib>:"Clear Errors.vi"("error in (no error)"=w351) -> ("error out"=w350:errorcluster)  [unwired: 5 in, 1 out]
        n132 = call <vilib>:"Open TCP Session.vi"("error in (no error)"=w350, "Port (502)"=u16 10, "IP Address"="localhost") -> ("error out"=w349:errorcluster, "MB_TCP session"=w354:refnum<class "MB_Master_TCP.lvclass">)  [unwired: 7 in]
        n133 = case shown="无错误" w349 {
          tunnel: w348 -> [w358 w359]
          tunnel: [w357 w359] -> w347
          frame No Error {
            n134 = Increment(x=w358) -> (x+1=w357:enum16{"open", "read", "write", "close"})
          }
          frame Error {
          }
        }
      }
      frame "read" {
        # "测量数据"
        n135 = call <vilib>:"Read Holding Registers.vi"("error in (no error)"=w365, "quantity"=u16 57, "starting address"=u16 0, "MB session in"=w368) -> ("error out"=w360:errorcluster, "Registers"=w363:u16[], "MB session out"=w361:refnum<class "MB_Master.lvclass">)  [unwired: 5 in]
        n136 = Array To Cluster(array=w363) -> (cluster=w362:T4)
        n137 = global write "与采配水交互全局.vi" "状态"(w362) -> ()
        n138 = case shown="错误" w360 {
          tunnel: [enum16{"open", "read", "write", "close"}."read" enum16{"open", "read", "write", "close"}."close"] -> w364
          frame No Error {
          }
          frame Error {
          }
        }
      }
      frame "write" {
        n139 = call <vilib>:"Write Multiple Registers.vi"("error in (no error)"=w375, "values"="values 6", "starting address"="starting address 6", "MB session in"=w376) -> ("error out"=w373:errorcluster, "MB session out"=w374:refnum<class "MB_Master.lvclass">)  [unwired: 6 in]
        n140 = case shown="错误" w373 {
          tunnel: [enum16{"open", "read", "write", "close"}."read" enum16{"open", "read", "write", "close"}."close"] -> w377
          frame No Error {
          }
          frame Error {
          }
        }
      }
      frame "close" {
        n141 = call-dynamic "Close Session.vi"("error in (no error)"=w383, "MB session in"=w384) -> ("error out"=w382:errorcluster)  [unwired: 9 in]
        n142 = call <vilib>:"Clear Errors.vi"("error in (no error)"=w382) -> ("error out"=w381:errorcluster)  [unwired: 5 in, 1 out]
      }
    }
  }
  n143 = while {
    tunnel: w3 -> [w392]
    tunnel: w2 -> [w401]
    tunnel: [w393] -> _
    shift-right: [w397] -> _
    shift-left: _ -> [w396]
    tunnel: errorcluster {"status"=FALSE, "code"=0, "source"=""} ("error out") -> [w395]
    tunnel: w4 -> [_]
    stop <- FALSE stop-if-true
    n144 = Get Queue Status(queue=w392) -> (queue out=w386:refnum<queue>, # pending insert=→"待处理插入数量":i32, error out=w385:errorcluster, # elements in queue=w389:i32, elements=→"元素":cluster{"命令":string}[])  [unwired: 2 in, 3 out]
    "队列中元素数量" <- w389
    n145 = Dequeue Element(queue=w392, error in (no error)=w401) -> (element=w400:cluster{"命令":string})  [unwired: 1 in, 3 out]
    n146 = Greater Or Equal?(x=w389, y=30) -> (x >= y?=w387:bool)
    n147 = case shown="真" w387 {
      tunnel: w386 -> [_ w404]
      tunnel: w385 -> [_ w403]
      frame False {
      }
      frame True {
        n148 = Flush Queue(queue=w404, error in (no error)=w403) -> ()  [unwired: 3 out]
      }
    }
    n149 = Unbundle By Name(w400) -> ("命令"=w399:string)
    n150 = case shown="\"氨氮读取\"" w399 {
      tunnel: [w406 w408 w418 w431 w443 w455 w467 w479] -> w397
      tunnel: [w405 w413 w420 w426 w437 w449 w461 w473] -> w393
      tunnel: w396 -> [w406 _ _ w429 w441 w453 w465 w477]
      tunnel: w395 -> [w405 w411 w421 w435 w447 w459 w471 w483]
      frame Default {
      }
      frame "启用模块" {
        n151 = global read "断电保存全局.vi" "MB通信方式选择"() -> (w407:enum16{"串口", "TCP"})
        n152 = call "质控单元MB_api.vi"("STEP"=enum16{"open", "read", "write", "close"}."open", "Error in"=w411) -> ("error out"=w413:errorcluster, "MB session out"=w409:refnum<class "MB_Master.lvclass">, "MB_TCP session"=w410:refnum<class "MB_Master_TCP.lvclass">)  [unwired: 6 in, 1 out]
        n153 = case shown="\"串口\", 默认" w407 {
          tunnel: w410 -> [_ w415]
          tunnel: w409 -> [w414 _]
          tunnel: [w414 w415] -> w408
          frame "串口", Default {
          }
          frame "TCP" {
          }
        }
      }
      frame "停用模块" {
        n154 = global read "断电保存全局.vi" "MB通信方式选择"() -> (w416:enum16{"串口", "TCP"})
        n155 = call "质控单元MB_api.vi"("STEP"=enum16{"open", "read", "write", "close"}."close", "Error in"=w421) -> ("error out"=w420:errorcluster, "MB session out"=w419:refnum<class "MB_Master.lvclass">, "MB_TCP session"=w417:refnum<class "MB_Master_TCP.lvclass">)  [unwired: 6 in, 1 out]
        n156 = case shown="\"串口\", 默认" w416 {
          tunnel: w417 -> [_ w424]
          tunnel: w419 -> [w423 _]
          tunnel: [w423 w424] -> w418
          frame "串口", Default {
          }
          frame "TCP" {
          }
        }
      }
      frame "氨氮读取" {
        n157 = property class="MB_Master"(reference=w429, "Properties:Slave ID"=u8 1 ("Slave ID")) -> (reference out=w428:refnum<class "MB_Master.lvclass">)  [unwired: 1 in, 1 out]
        n158 = call <vilib>:"Read Holding Registers.vi"("error in (no error)"=w435, "quantity"=u16 5 ("number of holding registers"), "starting address"=u16 100, "MB session in"=w428) -> ("error out"=w426:errorcluster, "Registers"=w432:u16[], "MB session out"=w431:refnum<class "MB_Master.lvclass">)  [unwired: 5 in]
        n159 = case shown="无错误" w426 {
          tunnel: w432 -> [w436 _]
          frame No Error {
            n160 = global write "质控内部交互全局.vi" "氨氮测量状态"(w436) -> ()
            "氨氮测量状态" <- w436
          }
          frame Error {
          }
        }
        n161 = Unbundle By Name(w426) -> ("status"=w427:bool)
        n162 = Not(x=w427) -> (.not. x?=w425:bool)
        n163 = global write "质控内部交互全局.vi" "氨氮通讯状态"(w425) -> ()
      }
      frame "总磷读取" {
        n164 = property class="MB_Master"(reference=w441, "Properties:Slave ID"=u8 2 ("Slave ID")) -> (reference out=w440:refnum<class "MB_Master.lvclass">)  [unwired: 1 in, 1 out]
        n165 = call <vilib>:"Read Holding Registers.vi"("error in (no error)"=w447, "quantity"=u16 5 ("number of holding registers"), "starting address"=u16 100, "MB session in"=w440) -> ("error out"=w437:errorcluster, "Registers"=w444:u16[], "MB session out"=w443:refnum<class "MB_Master.lvclass">)  [unwired: 5 in]
        n166 = case shown="无错误" w437 {
          tunnel: w444 -> [w448 _]
          frame No Error {
            n167 = global write "质控内部交互全局.vi" "总磷测量状态"(w448) -> ()
            "总磷测量状态" <- w448
          }
          frame Error {
          }
        }
        n168 = Unbundle By Name(w437) -> ("status"=w439:bool)
        n169 = Not(x=w439) -> (.not. x?=w438:bool)
        n170 = global write "质控内部交互全局.vi" "总磷通讯状态"(w438) -> ()
      }
      frame "总氮读取" {
        n171 = property class="MB_Master"(reference=w453, "Properties:Slave ID"=u8 2 ("Slave ID")) -> (reference out=w452:refnum<class "MB_Master.lvclass">)  [unwired: 1 in, 1 out]
        n172 = call <vilib>:"Read Holding Registers.vi"("error in (no error)"=w459, "quantity"=u16 5 ("number of holding registers"), "starting address"=u16 100, "MB session in"=w452) -> ("error out"=w449:errorcluster, "Registers"=w456:u16[], "MB session out"=w455:refnum<class "MB_Master.lvclass">)  [unwired: 5 in]
        n173 = case shown="无错误" w449 {
          tunnel: w456 -> [w460 _]
          frame No Error {
            n174 = global write "质控内部交互全局.vi" "总氮测量状态"(w460) -> ()
            "总氮测量状态" <- w460
          }
          frame Error {
          }
        }
        n175 = Unbundle By Name(w449) -> ("status"=w451:bool)
        n176 = Not(x=w451) -> (.not. x?=w450:bool)
        n177 = global write "质控内部交互全局.vi" "总氮通讯状态"(w450) -> ()
      }
      frame "CODMn读取" {
        n178 = property class="MB_Master"(reference=w465, "Properties:Slave ID"=u8 3 ("Slave ID")) -> (reference out=w464:refnum<class "MB_Master.lvclass">)  [unwired: 1 in, 1 out]
        n179 = call <vilib>:"Read Holding Registers.vi"("error in (no error)"=w471, "quantity"=u16 5 ("number of holding registers"), "starting address"=u16 100, "MB session in"=w464) -> ("error out"=w461:errorcluster, "Registers"=w468:u16[], "MB session out"=w467:refnum<class "MB_Master.lvclass">)  [unwired: 5 in]
        n180 = case shown="无错误" w461 {
          tunnel: w468 -> [w472 _]
          frame No Error {
            n181 = global write "质控内部交互全局.vi" "CODMn测量状态"(w472) -> ()
            "CODMn测量状态" <- w472
          }
          frame Error {
          }
        }
        n182 = Unbundle By Name(w461) -> ("status"=w463:bool)
        n183 = Not(x=w463) -> (.not. x?=w462:bool)
        n184 = global write "质控内部交互全局.vi" "CODMn通讯状态"(w462) -> ()
      }
      frame "CODCr读取" {
        n185 = property class="MB_Master"(reference=w477, "Properties:Slave ID"=u8 4 ("Slave ID")) -> (reference out=w476:refnum<class "MB_Master.lvclass">)  [unwired: 1 in, 1 out]
        n186 = call <vilib>:"Read Holding Registers.vi"("error in (no error)"=w483, "quantity"=u16 5 ("number of holding registers"), "starting address"=u16 100, "MB session in"=w476) -> ("error out"=w473:errorcluster, "Registers"=w480:u16[], "MB session out"=w479:refnum<class "MB_Master.lvclass">)  [unwired: 5 in]
        n187 = case shown="无错误" w473 {
          tunnel: w480 -> [w484 _]
          frame No Error {
            n188 = global write "质控内部交互全局.vi" "CODCr测量状态"(w484) -> ()
            "CODCr测量状态" <- w484
          }
          frame Error {
          }
        }
        n189 = Unbundle By Name(w473) -> ("status"=w475:bool)
        n190 = Not(x=w475) -> (.not. x?=w474:bool)
        n191 = global write "质控内部交互全局.vi" "CODCr通讯状态"(w474) -> ()
      }
    }
    n192 = Unbundle By Name(w393) -> ("status"=w398:bool)
    n193 = Not(x=w398) -> (.not. x?=→"通讯状态":bool)
  }
